vi "Publish.vi"(5 "Webpage Root":path, 6 "High Level Config Settings":T2={"Default Refresh Rate (ms)"=500, "Show Border"=FALSE, "Periodic Decoration Data"=FALSE, "Synchronous Requests"=FALSE, "Reduce Sent Data"=FALSE, "Recommended Control Settings"=TRUE}, 7 "VI Identifier":string, 9 "Host Connection":string="localhost", 10 "Default Control Behavior":T3, 11 "Config Option":T1) -> (0 "error out":errorcluster, 2 "Created JS":path, 3 "Created HTML":path)   [LabVIEW 2017, in "Front Panel Publisher.lvlib"]
doc: "This VI will initialize the FP Publisher code. To confure the settings, provide a true to <b>show Config Dialog</b>. \n\nThis dialog will also be shown if there are controls or indicators not yet configured. Settings for controls can be forced into one of three categories of Image, Value, and Value and Position. Controls that start with a specified string can be defaulted to one of these categories.\n\nThere is alos the <b>Host Connection</b> if this is unwired and localhost is used, then this webpage can only be access from this computer. Provide the external IP address to have access from other computers on the network."
uses:
  Front Panel Publisher.lvlib
  Web Front Panel_class/Controls/Cluster - Default Control Behavior.ctl
  Web Front Panel_class/Controls/High Level Config Settings.ctl
  Common/Enum - Config Option.ctl
  Front Panel Manager_class/Controls/Websocket Info.ctl
  Web Front Panel_class/Web Front Panel.lvclass
  Front Panel Manager_class/Front Panel Manager.lvclass
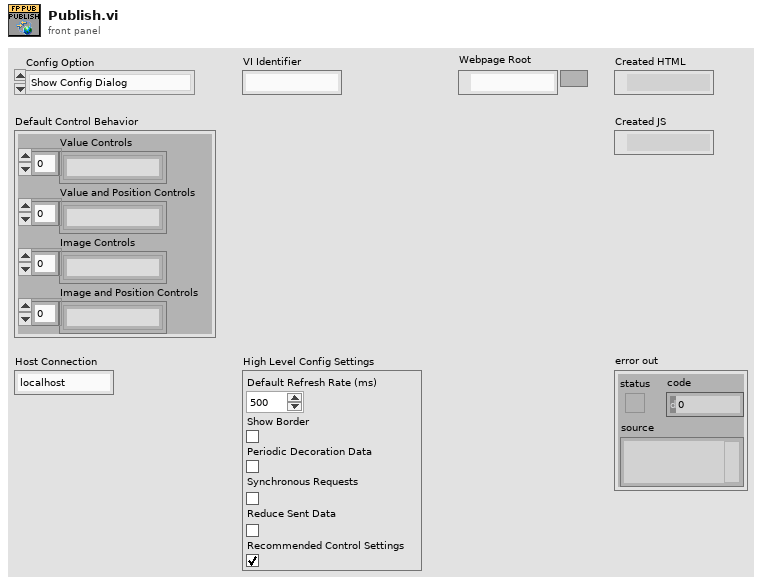
[diagram p1: front panel]
types:
  T1 = typedef "Front Panel Publisher.lvlib/Enum - Config Option.ctl" = enum16{"Show Config Dialog", "Don't Show Config Dialog", "Load Config File then Show Dialog", "Load Config File No Dialog"}
  T2 = typedef "Front Panel Publisher.lvlib/Web Front Panel.lvclass/High Level Config Settings.ctl" = cluster{"Default Refresh Rate (ms)":i32, "Show Border":bool, "Periodic Decoration Data":bool, "Synchronous Requests":bool, "Reduce Sent Data":bool, "Recommended Control Settings":bool}
  T3 = typedef "Front Panel Publisher.lvlib/Web Front Panel.lvclass/Cluster - Default Control Behavior.ctl" = cluster{"Value Controls":string[], "Value and Position Controls":string[], "Image Controls":string[], "Image and Position Controls":string[]}
  T4 = typedef "Front Panel Publisher.lvlib/Front Panel Manager.lvclass/Websocket Info.ctl" = cluster{"Hostname":string, "Port":u16}
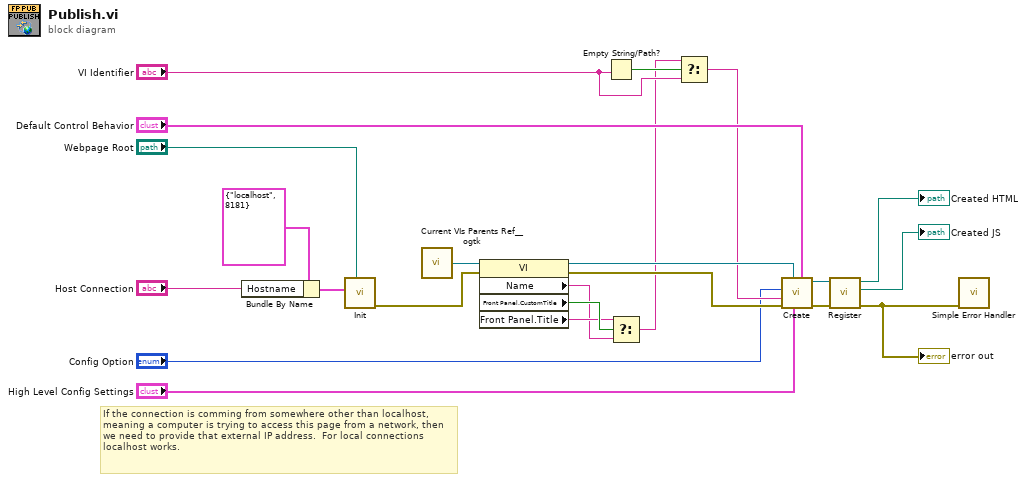
[diagram p0: block diagram]
diagram:
  # "If the connection is comming from somewhere other than localhost, meaning a computer is trying to access this page from a network, then we need to provide that external IP address.  For local connections localhost works."
  n1 = Bundle By Name(cluster=T4 {"Hostname"="localhost", "Port"=8181} ("Websocket Info"), "Hostname"="Host Connection") -> (w11:T4)
  n2 = call "Init.vi"("Webpage Root"="Webpage Root", "Connection Info"=w11) -> ("error out"=w19:errorcluster)  [unwired: 8 in, 1 out]
  n3 = call <userlib>:"Current VIs Parents Ref__ogtk.vi"() -> ("Calling VI's Reference"=w21:refnum<vi>)  [unwired: 2 in]
  n4 = property class="VI"(reference=w21, error in=w19) -> (reference out=w20:refnum<vi>, error out=w18:errorcluster, "Name"=w13:string, "Front Panel.CustomTitle"=w15:bool, "Front Panel.Title"=w14:string)
  n5 = Empty String/Path?(string/path="VI Identifier") -> (empty?=w7:bool)
  n6 = Select(t=w14, s=w15, f=w13) -> (s? t:f=w4:string)
  n7 = Select(t=w4, s=w7, f="VI Identifier") -> (s? t:f=w5:string)
  n8 = call "Create.vi"("Default Control Behavior"="Default Control Behavior", "High Level Config Settings"="High Level Config Settings", "VI Reference"=w20, "error in (no error)"=w18, "VI Name"=w5, "Config Option"="Config Option") -> ("error out"=w23:errorcluster, "Web FP Out"=w22:refnum<class "Web Front Panel.lvclass">)  [unwired: 4 in]
  n9 = call "Register.vi"("error in (no error)"=w23, "Web FP In"=w22) -> ("error out"=w17:errorcluster, "Created JS"=→"Created JS":path, "Created HTML"=→"Created HTML":path)  [unwired: 7 in]
  "error out" <- w17
  n10 = call <vilib>:"Simple Error Handler.vi"("error in (no error)"=w17) -> ()  [unwired: 4 in, 5 out]
